vi "Tosca-Flush IPC.vi"(7 "IPC":T1, 11 "error in (no error)":errorcluster) -> (15 "error out":errorcluster)   [LabVIEW 2020]
uses:
  Tosca-IPC.ctl
  Classes/Parameters/Parameters.lvclass
  Digital Input VIs/Tosca-DI Queue Data.ctl
  Digital Input VIs/Tosca-Input Event.ctl
  Digital Input VIs/Tosca-Input Criterion.ctl
  epl-vi-lib/Utility VIs/Type Defs/Logic State.ctl
  Typedefs/Tosca-Accumulator.ctl
  Typedefs/Tosca-State AODO.ctl
  Typedefs/Tosca-AO Runtime.ctl
  Typedefs/Tosca-DO Runtime.ctl
  epl-vi-lib/Signal Synthesis VIs/4th Generation/Classes/SignalManager/SignalManager.lvclass
  Typedefs/Tosca-Synapse Start Data.ctl
  Tosca-Message.ctl
  Tosca-Message Action.ctl
  Typedefs/Tosca-Thread Type.ctl
  Imaging VIs/Tosca-2P-Notifier Data.ctl
  Typedefs/Tosca-MATLAB Queue Data.ctl
  Visual Stim VIs/Tosca-Grating.ctl
  Visual Stim VIs/Tosca-Grating Type.ctl
  Typedefs/Tosca-File IO Notification.ctl
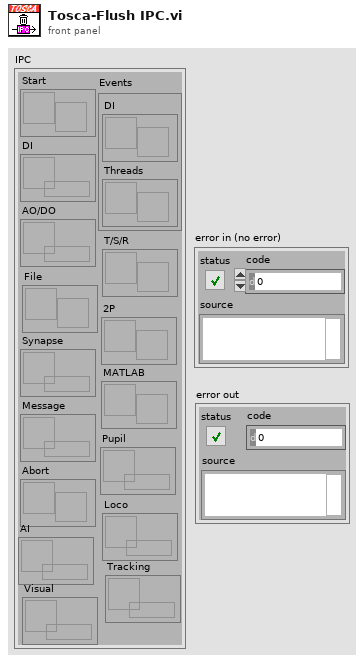
[diagram p1: front panel]
types:
  T1 = typedef "Tosca-IPC.ctl" = cluster{"Start":refnum<notifier>, "DI":refnum<queue>, "AO/DO":refnum<queue>, "Synapse":refnum<queue>, "Message":refnum<queue>, "Abort":refnum<notifier>, "Events":cluster{"DI":refnum<user-event>, "Threads ":refnum<user-event>}, "T/S/R":refnum<notifier>, "2P":refnum<notifier>, "MATLAB":refnum<notifier>, "Pupil":refnum<queue>, "Loco":refnum<queue>, "AI":refnum<queue>, "Tracking":refnum<queue>, "Visual":refnum<queue>, "File":refnum<notifier>}
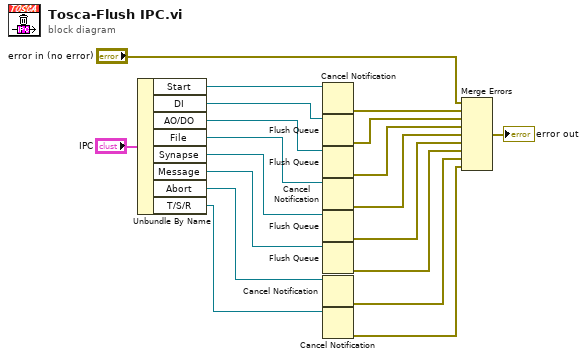
[diagram p0: block diagram]
diagram:
  n1 = Unbundle By Name("IPC") -> ("Start"=w13:refnum<notifier>, "DI"=w12:refnum<queue>, "AO/DO"=w11:refnum<queue>, "File"=w9:refnum<notifier>, "Synapse"=w10:refnum<queue>, "Message"=w7:refnum<queue>, "Abort"=w5:refnum<notifier>, "T/S/R"=w3:refnum<notifier>)
  n2 = Cancel Notification(0:w13) -> (11:w19:errorcluster)  [unwired: 1 in, 2 out]
  n3 = Flush Queue(queue=w12) -> (error out=w18:errorcluster)  [unwired: 1 in, 2 out]
  n4 = Flush Queue(queue=w11) -> (error out=w17:errorcluster)  [unwired: 1 in, 2 out]
  n5 = Cancel Notification(0:w9) -> (11:w8:errorcluster)  [unwired: 1 in, 2 out]
  n6 = Flush Queue(queue=w10) -> (error out=w16:errorcluster)  [unwired: 1 in, 2 out]
  n7 = Flush Queue(queue=w7) -> (error out=w6:errorcluster)  [unwired: 1 in, 2 out]
  n8 = Cancel Notification(0:w5) -> (11:w4:errorcluster)  [unwired: 1 in, 2 out]
  n9 = Cancel Notification(0:w3) -> (11:w2:errorcluster)  [unwired: 1 in, 2 out]
  n10 = Merge Errors("error in (no error)", w19, w18, w17, w8, w16, w6, w4, w2) -> (→"error out":errorcluster)
